vi "Get_Notebooks.vi"(8 "error in (no error)":errorcluster, 11 "Notebook in":refnum<class "Notebook.lvclass">) -> (0 "error out":errorcluster, 3 "Notebook out":refnum<class "Notebook.lvclass">)   [LabVIEW 2016, in "Notebook.lvclass"]
uses:
  Notebook.lvclass
  Object Oriented Version/Response/Response.lvclass
panel:
  out "Response Body":string
  out "Status Description":string
  out "Status Code":dbl
  in  "Authorization Code":string
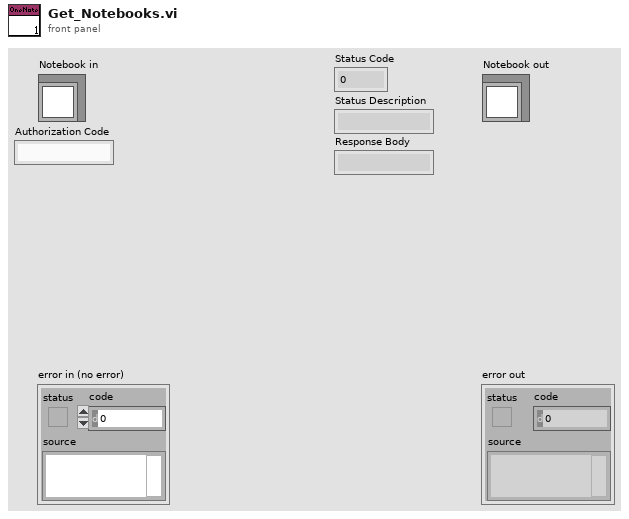
[diagram p1: front panel]
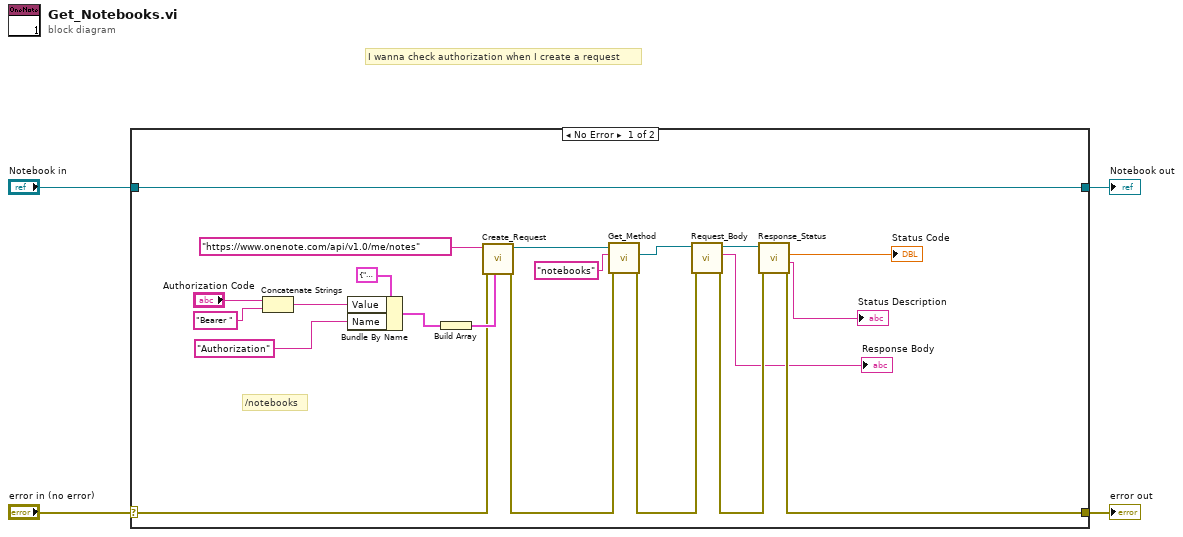
[diagram p0: block diagram]
diagram:
  # "I wanna check authorization when I create a request"
  n1 = case shown="No Error" "error in (no error)" {
    selector: "error in (no error)" -> [w7 w27]
    tunnel: [w6 w27] -> w3
    tunnel: [w25 w26] -> w1
    tunnel: "Notebook in" -> [w25 w26]
    frame No Error {
      # "/notebooks"
      n2 = Concatenate Strings("Authorization Code", "Bearer ") -> (w19:string)
      n3 = Bundle By Name(cluster=cluster{"Name":string, "Value":string} {"Name"="", "Value"=""} ("Header"), "Value"=w19, "Name"="Authorization") -> (w18:cluster{"Name":string, "Value":string})
      n4 = Build Array(w18) -> (w17:cluster{"Name":string, "Value":string}[])
      n5 = call "Create_Request.vi"("Headers"=w17, "error in (no error)"=w7, "Base URL"="https://www.onenote.com/api/v1.0/me/notes") -> ("error out"=w14:errorcluster, "Request out"=w16:refnum<class "Request.lvclass">)  [unwired: 7 in]
      n6 = call "Get_Method.vi"("error in (no error)"=w14, "Endpoint URL"="notebooks", "Request in"=w16) -> ("error out"=w12:errorcluster, "Response out"=w13:refnum<class "Response.lvclass">)  [unwired: 6 in, 1 out]
      n7 = call "Request_Body.vi"("error in (no error)"=w12, "Response in"=w13) -> ("error out"=w10:errorcluster, "Response Body"=→"Response Body":string, "Response out"=w11:refnum<class "Response.lvclass">)  [unwired: 7 in]
      n8 = call "Response_Status.vi"("error in (no error)"=w10, "Response in"=w11) -> ("error out"=w6:errorcluster, "Status Description"=→"Status Description":string, "Status Code"=→"Status Code":dbl)  [unwired: 6 in, 1 out]
    }
    frame Error {
    }
  }
  "error out" <- w3
  "Notebook out" <- w1
